vi "[SubVI]Reading_Right_LUT.vi"(11 "Input CSV":dbl[][](array[numeric])) -> (1 "Theta LUT":dbl[](array[numeric]), 3 "X LUT":dbl[](array[numeric]))   [LabVIEW 2017]
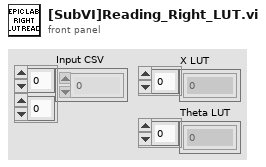
[diagram p1: front panel]
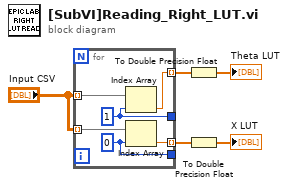
[diagram p0: block diagram]
diagram:
  n1 = for {
    tunnel: "Input CSV" -> [w11] mode=indexing
    tunnel: "Input CSV" -> [w10] mode=indexing
    tunnel: [w9] -> _
    tunnel: [w8] -> _
    tunnel: [w7] -> w4 mode=indexing
    tunnel: [w6] -> w2 mode=indexing
    w8 = 1 ("index")
    w9 = 0 ("index")
    n2 = Index Array(array=w10, index=w8) -> (element=w6:dbl)
    n3 = Index Array(array=w11, index=w9) -> (element=w7:dbl)
  }
  n4 = To Double Precision Float(number=w2) -> (double precision float=→"Theta LUT":dbl[])
  n5 = To Double Precision Float(number=w4) -> (double precision float=→"X LUT":dbl[])
